vi "Dictionary to Plot Names.vi"(8 "error in (no error)":errorcluster, 11 "Results (Dictionary)":cluster{"key":string, "value":dbl}[](array[cluster])) -> (0 "error out":errorcluster, 2 "Plot Names":string[](array[string]), 3 "Results (Dictionary) out":cluster{"key":string, "value":dbl}[](array[cluster]))   [LabVIEW 2019, in "Instrument.Lockin.lvlib" / "Instrument UI.Lockin.lvclass"]
uses:
  Instrument UI.Lockin.lvclass
  Instrument.Lockin/Typedefs/Results Type--Enum.ctl
  Instrument.Lockin/Instrument.Lockin.lvclass
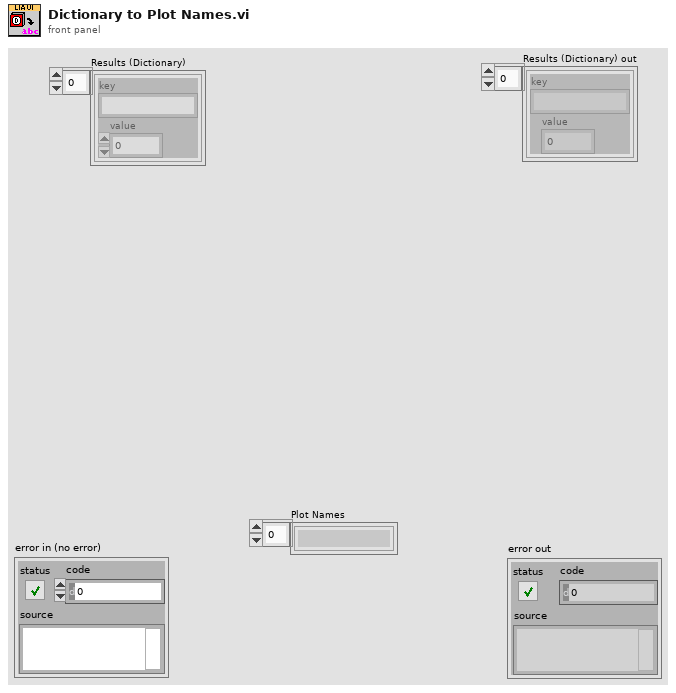
[diagram p1: front panel]
types:
  T1 = typedef "Instrument.Lockin.lvlib/Instrument.Lockin.lvclass/Results Type--Enum.ctl" = enum16{"X", "Y", "R", "Theta", "Mean"}
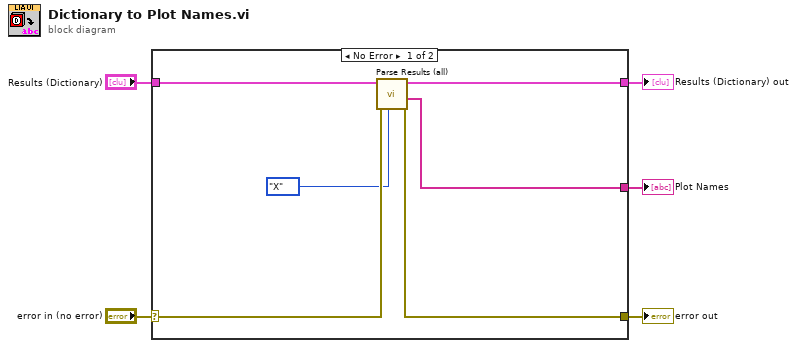
[diagram p0: block diagram]
diagram:
  n1 = case shown="No Error" "error in (no error)" {
    selector: "error in (no error)" -> [w7 w12]
    tunnel: "Results (Dictionary)" -> [w11 _]
    tunnel: [w8 w12] -> w3
    tunnel: [w10 _] -> w2
    tunnel: [w9 _] -> w1
    frame No Error {
      n2 = call "Parse Results (all).vi"("Type"=Results_Type--Enum."X", "error in (no error)"=w7, "Results (Dictionary)"=w11) -> ("error out"=w8:errorcluster, "Names"=w10:string[], "Results (Dictionary)"=w9:cluster{"key":string, "value":dbl}[])  [unwired: 5 in, 1 out]
    }
    frame Error {
    }
  }
  "error out" <- w3
  "Plot Names" <- w2
  "Results (Dictionary) out" <- w1
